vi "Read SessionType Property.vi"(8 "error in":errorcluster, 11 "port node in":refnum<k20>) -> (0 "error out":errorcluster, 2 "session type":string, 3 "port node out":refnum<k20>)   [LabVIEW 2020, in "AIM ARINC 664 Import.lvlib"]
uses:
  AIM ARINC 664 Import.lvlib
  <resource>/objmgr/DOMUserDefRef.rc
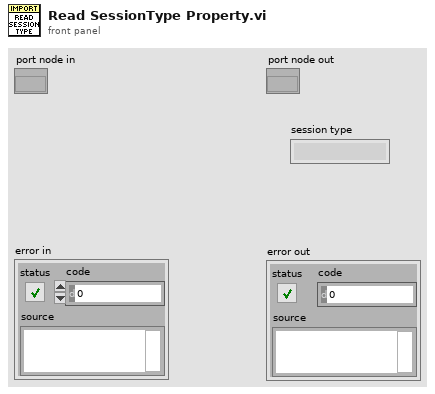
[diagram p1: front panel]
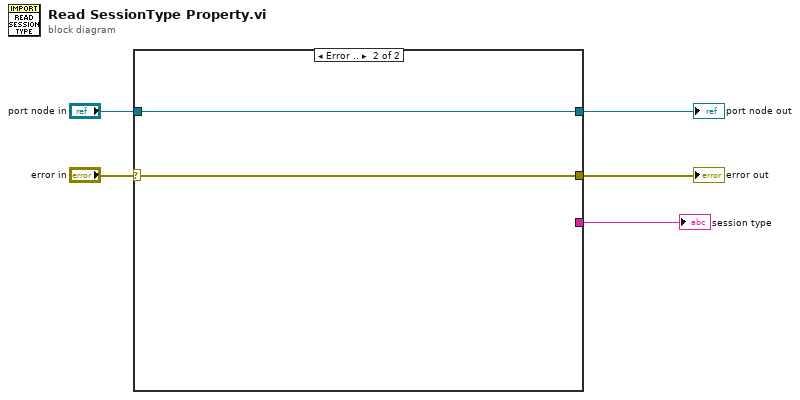
[diagram p0: block diagram]
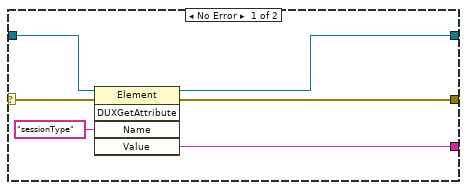
[diagram p2: hidden frame]
diagram:
  n1 = case shown="Error .." "error in" {
    selector: "error in" -> [w8 w13]
    tunnel: [w11 w13] -> w5
    tunnel: "port node in" -> [w10 w12]
    tunnel: [w9 w12] -> w3
    tunnel: [w6 _] -> w1
    frame No Error {
      n2 = invoke class="Element" method="DUXGetAttribute"(reference=w10, error in=w8, "Name"="sessionType") -> (reference out=w9:refnum<k20>, error out=w11:errorcluster, "Value"=w6:string)  [unwired: 2 in, 2 out]
    }
    frame Error {
    }
  }
  "error out" <- w5
  "port node out" <- w3
  "session type" <- w1
